vi "StateDiagramGraph_GetAttributes.vi"(0 "reference in":refnum<class "StateDiagramGraph.lvclass">, 5 "error in (no error)":errorcluster) -> (14 "reference out":refnum<class "StateDiagramGraph.lvclass">, 16 "Attributes":T1={"Base class"={"nodes"=[], "edges"=[], "nodesToBeRemoved"=[], "edgesToBeRemoved"=[], "needsLayout"=FALSE, "LayoutNodes"=[]}, "StateDiagramData"={"VI-Path"=path "", "ShowOption"=enum."Show Relative Path"}}, 17 "Attributes locked?":bool, 19 "error out":errorcluster)   [LabVIEW 2014, in "StateDiagramGraph.lvclass"]
doc: "Returns the attributes of a StateDiagramGraph object.\n\nIf the object is currently locked for modification, 'Attributes locked?' will return TRUE.\n\n[GOOP 2.0.15]"
uses:
  <resource>/Framework/Providers/Open_GDS/UML/StateDiagramGraph_class/StateDiagramGraph.lvclass
  <resource>/Framework/Providers/Open_GDS/UML/StateDiagramGraph_class/protected/ObjectAttributes.ctl
  <resource>/Framework/Providers/Open_GDS/UML/Graph_class/protected/ObjectAttributes.ctl
  <resource>/Framework/Providers/Open_GDS/UML/AbstractNode_class/AbstractNode.lvclass
  <resource>/Framework/Providers/Open_GDS/UML/AbstractEdge_class/AbstractEdge.lvclass
  <resource>/Framework/Providers/Open_GDS/UML/StateDiagramGraph_class/private/StateDiagramData.ctl
  <resource>/Framework/Providers/Open_GDS/UML/StateDiagramGraph_class/private/ViPathShowOption.ctl
  <vilib>/addons/_goop3.llb/3GOOPStates.ctl
  <resource>/Framework/Providers/Open_GDS/UML/StateDiagramGraph_class/StateDiagramGraph.lvclass/StateDiagramGraph.ctl
  <resource>/Framework/Providers/Open_GDS/UML/Graph_class/Graph.lvclass
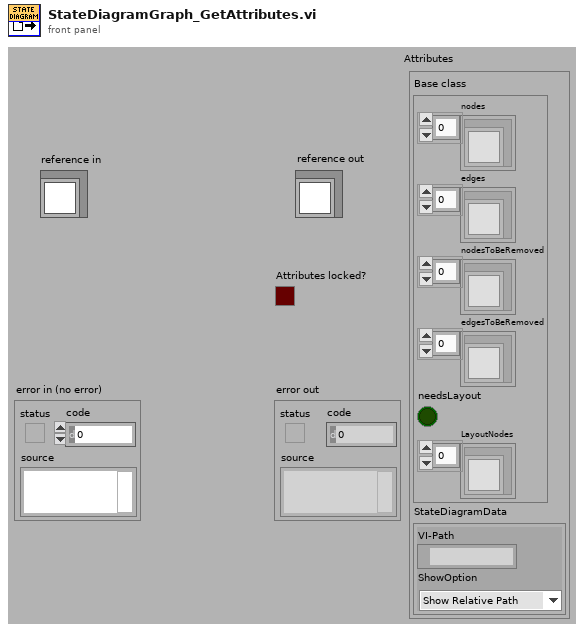
[diagram p1: front panel]
types:
  T1 = typedef "StateDiagramGraph.lvclass/ObjectAttributes.ctl" = cluster{"Base class":T2, "StateDiagramData":T3}
  T2 = typedef "Graph.lvclass/ObjectAttributes.ctl" = cluster{"nodes":refnum<class "AbstractNode.lvclass">[], "edges":refnum<class "AbstractEdge.lvclass">[], "nodesToBeRemoved":refnum<class "AbstractNode.lvclass">[], "edgesToBeRemoved":refnum<class "AbstractEdge.lvclass">[], "needsLayout":bool, "LayoutNodes":refnum<class "AbstractNode.lvclass">[]}
  T3 = typedef "StateDiagramGraph.lvclass/StateDiagramData.ctl" = cluster{"VI-Path":path, "ShowOption":T4}
  T4 = typedef "StateDiagramGraph.lvclass/ViPathShowOption.ctl" = enum16{"Don't Show", "Show Relative Path", "Show Absolute Path"}
  T5 = typedef "3GOOPStates.ctl" = enum16{"Set", "Get", "New", "Delete", "Clear", "Test and get", "Unlock data", "Information", "Look up existing", "New or look up existing", "Test and get shared", "Get shared", "Set shared", "Unlock shared", "Find dynamic method", "Register dynamic method", "Preload dynamic method", "Probe", "Cast to more generic", "Cast to more specific"}
  T6 = typedef "Graph.lvclass/ObjectReference.ctl" = refnum<k1>
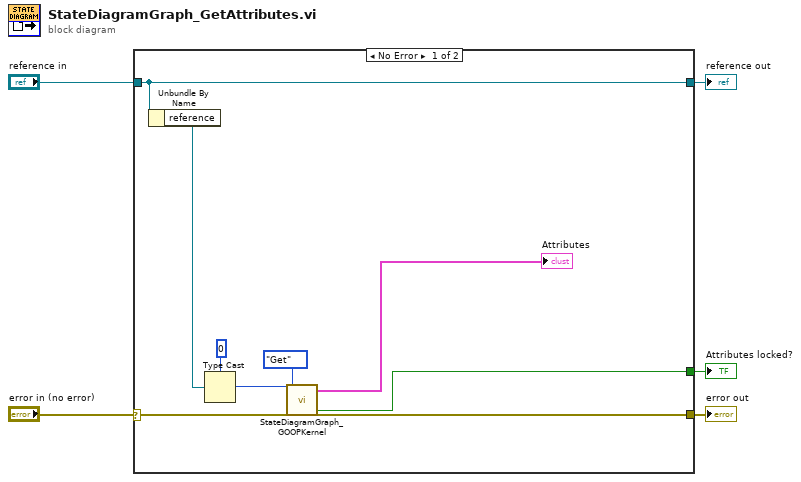
[diagram p0: block diagram]
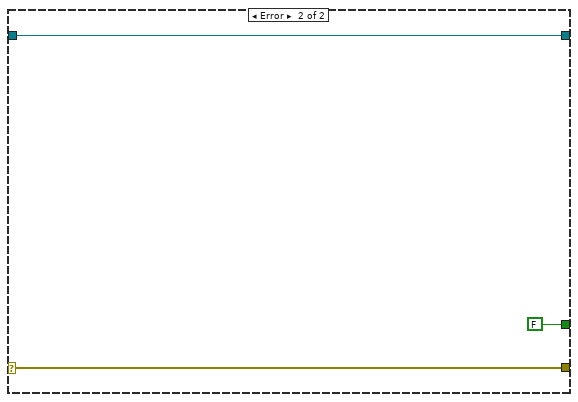
[diagram p2: hidden frame]
diagram:
  n1 = case shown="No Error" "error in (no error)" {
    selector: "error in (no error)" -> [w13 w16]
    tunnel: [w7 w17] -> w5
    tunnel: [w11 w16] -> w4
    tunnel: "reference in" -> [w7 w17]
    tunnel: [w10 FALSE ("Data locked?")] -> w1
    frame No Error {
      n2 = Unbundle By Name(w7) -> ("reference"=w6:T6)
      n3 = Type Cast(type=0, x=w6) -> (*(type *) &x=w12:i32)
      n4 = call <resource>:"StateDiagramGraph_GOOPKernel.vi"("Ref in"=w12, "error in (no error)"=w13, "Action"=3GOOPStates."Get") -> ("Data out"=→"Attributes":T1, "Data locked?"=w10:bool, "error out"=w11:errorcluster)  [unwired: 12 in, 10 out]
    }
    frame Error {
    }
  }
  "error out" <- w4
  "reference out" <- w5
  "Attributes locked?" <- w1
